vi "Format Bond Pad Points.vi"(4 "WorkTable":refnum<class "WorkTable Class.lvclass">, 6 "Bond Pad Groups":T2[](array[typedef]), 7 "Part Type":T1, 8 "error in":errorcluster, 9 "Slot":i32, 10 "Chuck":i32, 11 "Console Log in":refnum<class "Console Log.lvclass">) -> (0 "error out":errorcluster, 2 "Formatted Bond Pads":string[](array[string]), 3 "Console Log out":refnum<class "Console Log.lvclass">)   [LabVIEW 2011, in "Console Log.lvclass"]
uses:
  Console Log.lvclass
  Shared Components/Utils/Type Definitions/3d Line.ctl
  Shared Components/Vec3d Class/Vec3d Class.lvclass
  Shared Components/Config Manager Class/Type Definitions/Part Type.ctl
  Shared Components/WorkTable Class/WorkTable Class.lvclass
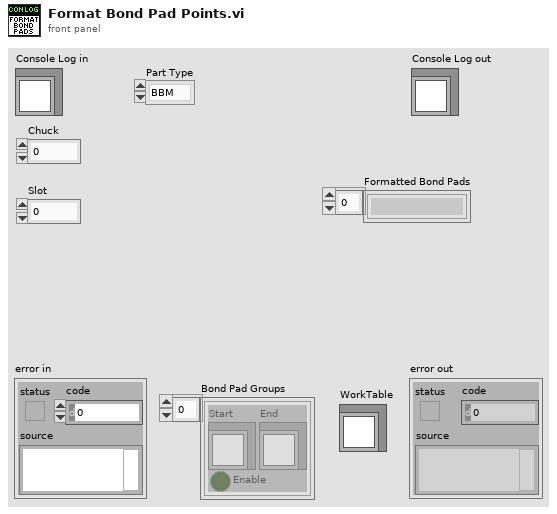
[diagram p1: front panel]
types:
  T1 = typedef "Part Type.ctl" = enum16{"BBM", "HDI", "BARE HDI", "GLUERESERVOIR", "STAMP_1", "STAMP_2", "STAMP_3", "STAMP_4", "STAMP_5", "WEIGHT_1", "WEIGHT_2", "WEIGHT_3", "WEIGHT_4", "WEIGHT_5", "WEIGHT_6", "WEIGHT_7", "WEIGHT_8", "PICKER_TOOL", "GRABER_TOOL"}
  T2 = typedef "3d Line.ctl" = cluster{"Start":refnum<class "Vec3d Class.lvclass">, "End":refnum<class "Vec3d Class.lvclass">, "Enable":bool}
  T3 = typedef "Worktable_Module Slot.ctl" = cluster{"Slot State":enum16{"Empty", "Bare HDI", "Unglued", "Stamped", "PartOnTop", "Weighted", "Unpotted", "Potted"}, "BBM Type":enum16{"None", "BBM", "GlassSlide"}, "HDI Type":enum16{"None", "HDI", "Polyimide"}, "Vacuum Channel":u8, "Location/Orientation BBM":T4, "Location/Orientation HDI":T4, "S/N":string}
  T4 = typedef "Position_Orientation.ctl" = cluster{"Center":refnum<class "Vec3d Class.lvclass">, "Orientation":refnum<class "Orient3d Class.lvclass">}
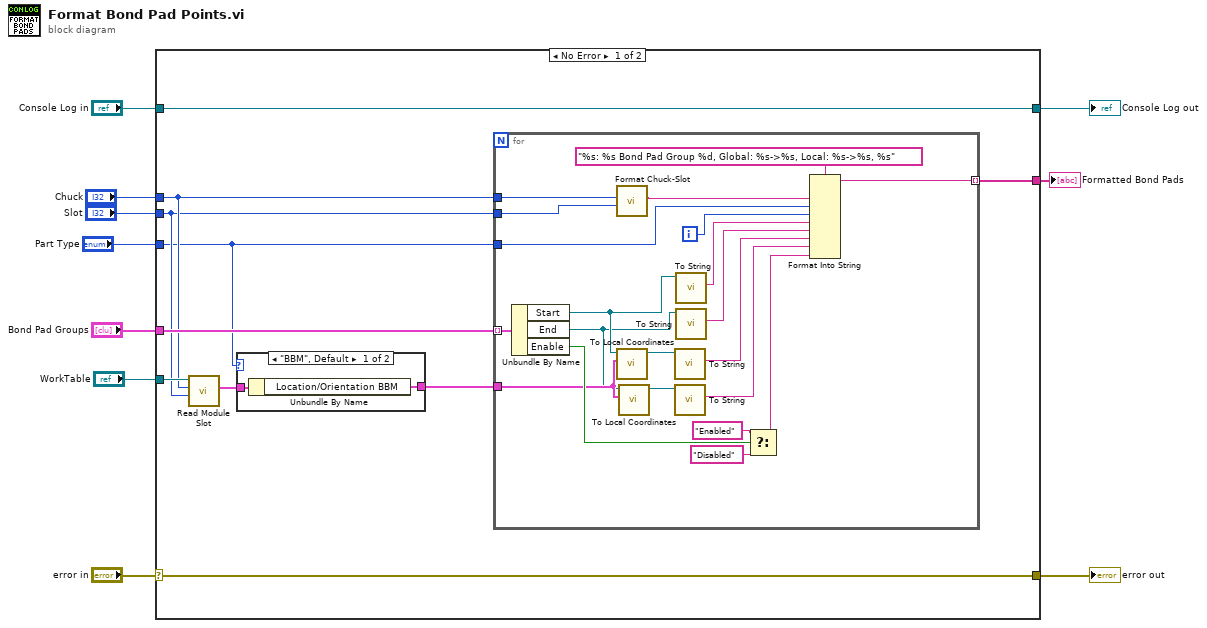
[diagram p0: block diagram]
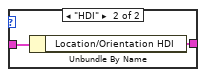
[diagram p2: hidden frame]
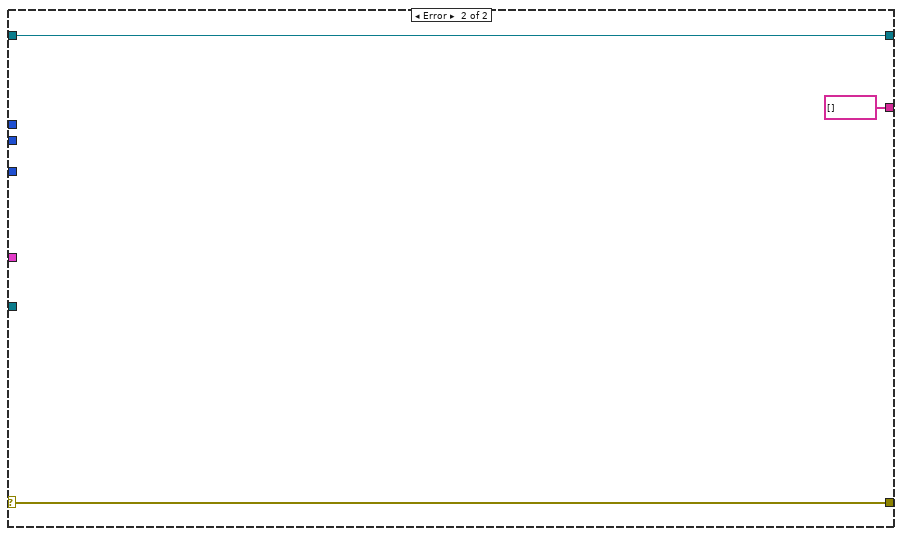
[diagram p3: hidden frame]
diagram:
  n1 = case shown="No Error" "error in" {
    selector: "error in" -> [w19 w48]
    tunnel: [w19 w48] -> w9
    tunnel: [w20 w47] -> w7
    tunnel: "Console Log in" -> [w20 w47]
    tunnel: "Bond Pad Groups" -> [w18 _]
    tunnel: [w17 string[] []] -> w5
    tunnel: "Chuck" -> [w15 _]
    tunnel: "Slot" -> [w14 _]
    tunnel: "WorkTable" -> [w16 _]
    tunnel: "Part Type" -> [w12 _]
    frame No Error {
      n2 = call-dynamic "Read Module Slot.vi"("slot"=w14, "chuck"=w15, "WorkTable in"=w16) -> ("Module Slot"=w13:T3)  [unwired: 6 in, 2 out]
      n3 = case shown="\"BBM\", Default" w12 {
        tunnel: w13 -> [w22 w24]
        tunnel: [w21 w23] -> w11
        frame "BBM", Default {
          n4 = Unbundle By Name(w22) -> ("Location/Orientation BBM"=w21:T4)
        }
        frame "HDI" {
          n5 = Unbundle By Name(w24) -> ("Location/Orientation HDI"=w23:T4)
        }
      }
      n6 = for {
        tunnel: w18 -> [w45] mode=indexing
        tunnel: [w37] -> w17 mode=indexing
        tunnel: w15 -> [w34]
        tunnel: w14 -> [w33]
        tunnel: w12 -> [w32]
        tunnel: w11 -> [w31]
        i -> [w40]
        n7 = Unbundle By Name(w45) -> ("Start"=w30:refnum<class "Vec3d Class.lvclass">, "End"=w29:refnum<class "Vec3d Class.lvclass">, "Enable"=w44:bool)
        n8 = call "Format Chuck-Slot.vi"("Slot"=w33, "Chuck"=w34) -> ("Formatted Chuck/Slot"=w36:string)  [unwired: 7 in, 2 out]
        n9 = call "To Local Coordinates.vi"("Center/Orientation"=w31, "Global Coordinates"=w30) -> ("Local Coordinates"=w28:refnum<class "Vec3d Class.lvclass">)  [unwired: 8 in, 1 out]
        n10 = call "To Local Coordinates.vi"("Center/Orientation"=w31, "Global Coordinates"=w29) -> ("Local Coordinates"=w27:refnum<class "Vec3d Class.lvclass">)  [unwired: 8 in, 1 out]
        n11 = call "To String.vi"("Vec3d in"=w28) -> ("Vec3d String"=w26:string)  [unwired: 8 in, 2 out]
        n12 = call "To String.vi"("Vec3d in"=w27) -> ("Vec3d String"=w25:string)  [unwired: 8 in, 2 out]
        n13 = call "To String.vi"("Vec3d in"=w30) -> ("Vec3d String"=w39:string)  [unwired: 8 in, 2 out]
        n14 = call "To String.vi"("Vec3d in"=w29) -> ("Vec3d String"=w38:string)  [unwired: 8 in, 2 out]
        n15 = Select(t="Enabled", s=w44, f="Disabled") -> (s? t:f=w35:string)
        n16 = Format Into String(format string="%s: %s Bond Pad Group %d, Global: %s->%s, Local: %s->%s, %s", w36, w32, w40, w39, w38, w26, w25, w35) -> (resulting string=w37:string)  [unwired: 2 in, 1 out]
      }
    }
    frame Error {
    }
  }
  "error out" <- w9
  "Console Log out" <- w7
  "Formatted Bond Pads" <- w5
